vi "GetFrontPanelImage.vi"(8 "ErrorIn":errorcluster, 11 "ObjectIn":refnum<class "FrontPanelControl.lvclass">) -> (0 "ErrorOut":errorcluster, 2 "FPImage":picture, 3 "ObjectOut":refnum<class "FrontPanelControl.lvclass">)   [LabVIEW 2021, in "FrontPanelControl.lvclass"]
uses:
  FrontPanelControl.lvclass
  FrontPanelControl.lvclass/FrontPanelControl.ctl
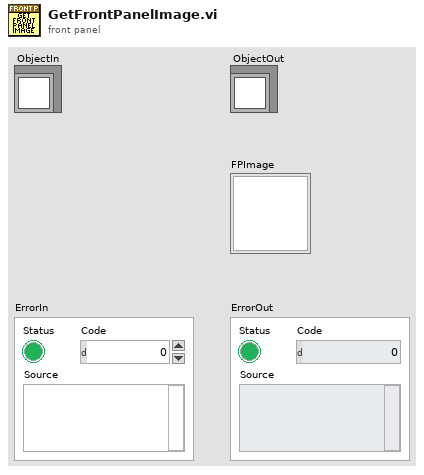
[diagram p1: front panel]
types:
  T1 = typedef "imagedata.ctl" = cluster{"image type":i32, "image depth":i32, "image":u8[], "mask":u8[], "colors":u32[], "Rectangle":cluster{"left":i16, "top":i16, "right":i16, "bottom":i16}}
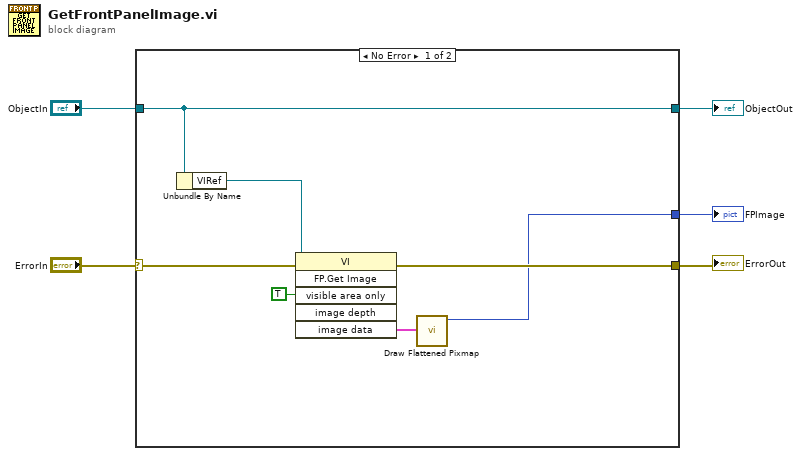
[diagram p0: block diagram]
diagram:
  n1 = case shown="No Error" "ErrorIn" {
    selector: "ErrorIn" -> [w12 w14]
    tunnel: [w11 w14] -> w4
    tunnel: [w10 w13] -> w2
    tunnel: "ObjectIn" -> [w10 w13]
    tunnel: [w6 _] -> w1
    frame No Error {
      n2 = Unbundle By Name(w10) -> ("VIRef"=w9:refnum<vi>)
      n3 = invoke class="VI" method="FP.Get Image"(reference=w9, error in=w12, "visible area only"=TRUE ("Visible Area Only")) -> (error out=w11:errorcluster, "image data"=w7:T1)  [unwired: 3 in, 4 out]
      n4 = call <vilib>:"Draw Flattened Pixmap.vi"("image data"=w7) -> ("new picture"=w6:picture)  [unwired: 8 in]
    }
    frame Error {
    }
  }
  "ErrorOut" <- w4
  "ObjectOut" <- w2
  "FPImage" <- w1
